vi "Open Solver.vi"(8 "error in (no error)":errorcluster, 11 "Solver Path":path) -> (0 "error IO":errorcluster, 2 "Scorer Context":refnum<vi>, 3 "Solver VI":T1)   [LabVIEW 2024, in "Wordle Scorer.lvlib"]
uses:
  Wordle Scorer.lvlib
  Solver VI Ref Type.ctl
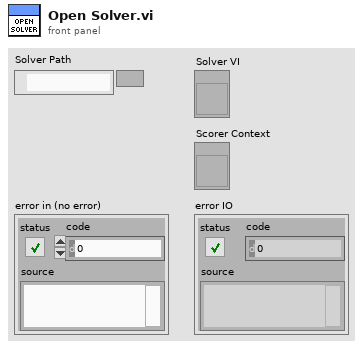
[diagram p1: front panel]
types:
  T1 = typedef "Wordle Scorer.lvlib/Solver VI Ref Type.ctl" = refnum<vi>
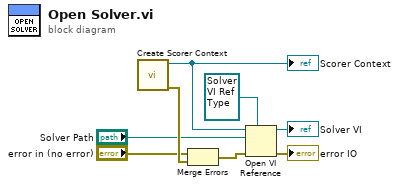
[diagram p0: block diagram]
diagram:
  n1 = call "Create Scorer Context.vi"() -> ("error out"=w8:errorcluster, "Scorer Context"=w1:refnum<vi>)  [unwired: 10 in]
  "Scorer Context" <- w1
  n2 = Merge Errors("error in (no error)", w8) -> (w2:errorcluster)
  n3 = Open VI Reference(type specifier VI Refnum (for type only)=T1 refnum ("Solver VI"), application reference (local)=w1, vi path="Solver Path", error in (no error)=w2) -> (vi reference=→"Solver VI":T1, error out=→"error IO":errorcluster)  [unwired: 2 in]
